vi "SEK2020v1VI5SeguirTubulacao.vi"(8 "Parâmetros":T1={"Azul Max EV3 Cor"=17, "Azul Min EV3 Cor"=0, "Verde Max EV3 Cor"=6, "Verde Min EV3 Cor"=0, "Vermelho Max Ev3 Cor"=0, "Vermelho Min EV3 Cor"=0, "Chão EV3 Cor"=0.0, "Branco Max EV3 Cor"=0.0, "Branco Min EV3 Cor"=0.0, "Preto Max EV3 Cor"=0.0, "Preto Min EV3 Cor"=0.0, "Distância Tubulação"=0.0, "Distância Frontal"=0.0, "Amarelo Max EV3 Cor"=0.0, "Amarelo Min EV3 Cor"=0.0, "Distância Lateral"=0.0, "90°"=0.0, "180°"=0.0, "Seguidor de Linha"=0.0}, 10 "NXT/EV3":T2) -> (1 "Boolean":bool, 2 "d-e":i32, 3 "NXT/EV3 2":T2)   [LabVIEW 2016]
uses:
  <vilib>/NXT/Subs/LVHSConnector.ctl
  <vilib>/NXT/LegoClasses/BrickReference/BrickReference.lvclass
  <vilib>/NXT/Block Support/NXT_OutputPort.ctl
  <vilib>/NXT/Block Support/NXT_InputPort.ctl
  <vilib>/NXT/Dual Mode Library/Sensors/EV3_Ultrasonic_CM.vi
  <vilib>/NXT/Dual Mode Library/Sensors/Touch_Pressed.vi
  <vilib>/NXT/NXTIO Xnodes/NXTIONodeSubVIs/NXTMoveMotors.vi
  <vilib>/NXT/NXTIO Xnodes/NXTIONodeSubVIs/NXTStopMotors.vi
  <vilib>/NXT/Dual Mode Library/Sensors/EV3_Color_Reflect.vi
  <vilib>/NXT/NXTIO Xnodes/AddressXNode/NXTIOAddress.xnode
  <vilib>/NXT/NXTIO Xnodes/NXTIOXNode/NXTIO.xnode
panel:
  # "Sensor EV3 Cor"
  # "Sensor Ultrassônico"
  # "Sensor Giroscópio"
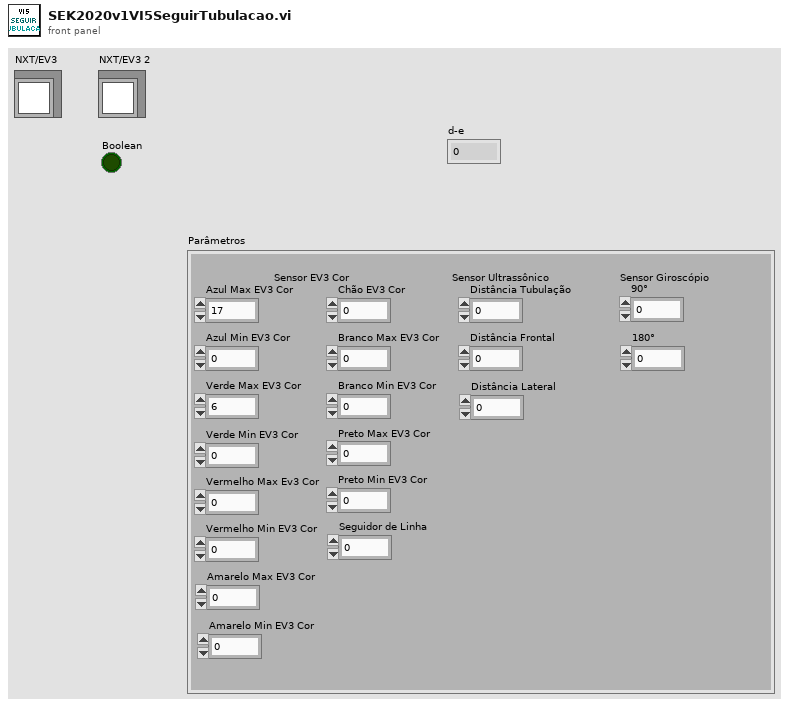
[diagram p1: front panel]
types:
  T1 = cluster{"Azul Max EV3 Cor":i32, "Azul Min EV3 Cor":i32, "Verde Max EV3 Cor":i32, "Verde Min EV3 Cor":i32, "Vermelho Max Ev3 Cor":i32, "Vermelho Min EV3 Cor":i32, "Chão EV3 Cor":sgl, "Branco Max EV3 Cor":sgl, "Branco Min EV3 Cor":sgl, "Preto Max EV3 Cor":sgl, "Preto Min EV3 Cor":sgl, "Distância Tubulação":sgl, "Distância Frontal":sgl, "Amarelo Max EV3 Cor":dbl, "Amarelo Min EV3 Cor":dbl, "Distância Lateral":sgl, "90°":sgl, "180°":sgl, "Seguidor de Linha":dbl}
  T2 = typedef "LVHSConnector.ctl" = refnum<class "BrickReference.lvclass">
  T3 = typedef "NXT_OutputPort.ctl" = u8
  T4 = typedef "NXT_InputPort.ctl" = u32
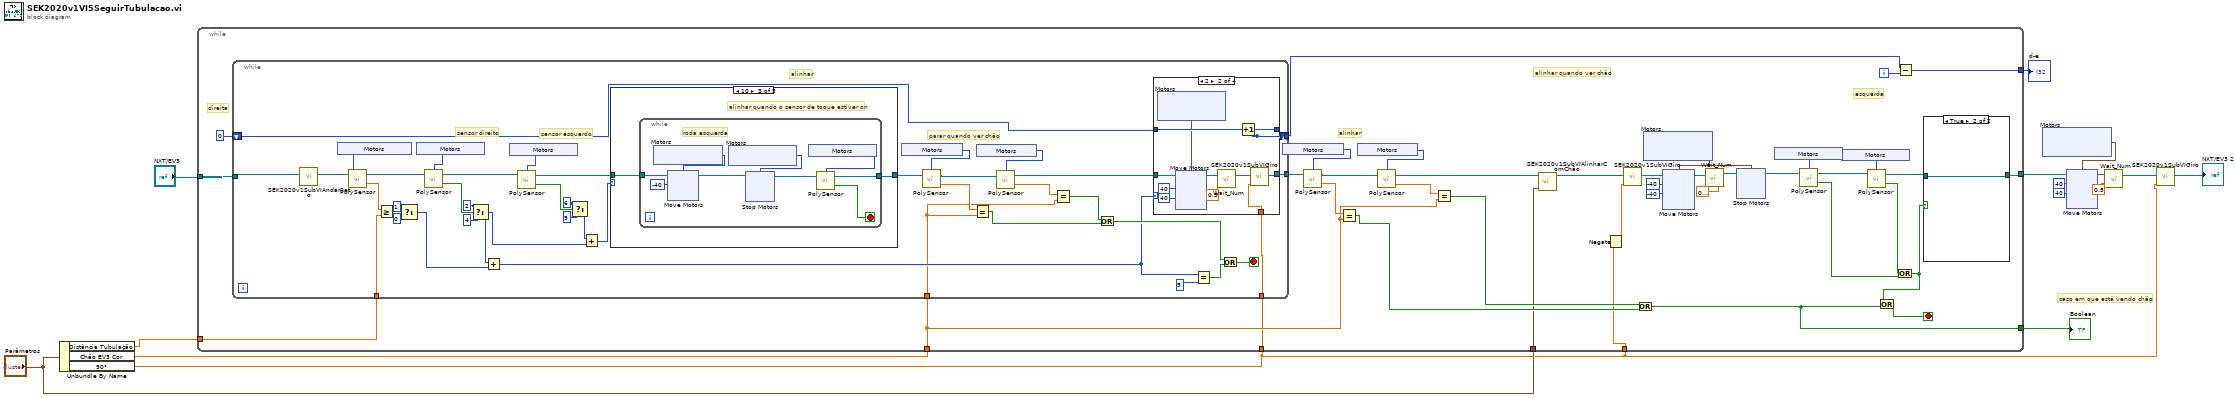
[diagram p0: block diagram]
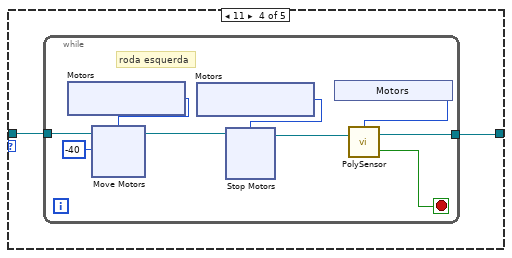
[diagram p4: hidden frame]
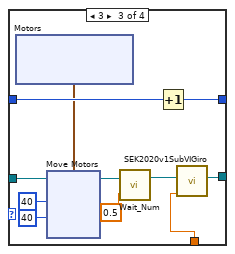
[diagram p7: hidden frame]
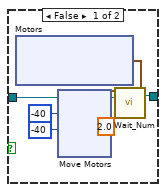
[diagram p9: hidden frame]
diagram:
  # "caso em que está vendo chão"
  n1 = Unbundle By Name("Parâmetros") -> ("Distância Tubulação"=w2:sgl, "Chão EV3 Cor"=w15:sgl, "90°"=w1:sgl)
  n2 = while {
    tunnel: "NXT/EV3" -> [w54]
    tunnel: [w33] -> w6
    tunnel: w15 -> [w39]
    tunnel: [w27] -> w13
    tunnel: [w35] -> w4
    tunnel: "Parâmetros" -> [w20]
    tunnel: w1 -> [w19]
    tunnel: w2 -> [w18]
    tunnel: w1 -> [w17]
    i -> [w37]
    stop <- w25 stop-if-true
    # "alinhar quando ver chão"
    # "esquerda"
    # "direita"
    # "alinhar"
    n3 = while {
      tunnel: w54 -> [w62]
      tunnel: [w83] -> w40
      tunnel: w39 -> [w59]
      tunnel: [w64] -> _
      shift-right: [w64] -> w36
      shift-left: 0 -> [w65]
      tunnel: w19 -> [w56]
      tunnel: w18 -> [w55]
      stop <- w66 stop-if-true
      # "parar quando ver chão"
      # "alinhar"
      # "sensor esquerdo"
      # "sensor direito"
      n4 = call "SEK2020v1SubVIAndarReto.vi"("NXT/EV3"=w62) -> ("NXT/EV3 2"=w96:T2)  [unwired: 9 in]
      n5 = xnode "Motors"() -> ("Sensor"=w95:T4)
      n6 = call-poly <vilib>:"PolySensor.vi"("NXT/EV3"=w96, "Port (Port 1)"=w95) -> ("Centimeters"=w92:sgl, "NXT/EV3"=w94:T2)  [unwired: 1 in]
      n7 = Greater Or Equal?(x=w92, y=w55) -> (x >= y?=w91:bool)
      n8 = Select(t=1, s=w91, f=0) -> (s? t:f=w85:i32)
      n9 = xnode "Motors"() -> ("Sensor"=w93:T4)
      n10 = call-poly <vilib>:"PolySensor.vi"("NXT/EV3"=w94, "Port (Port 1)"=w93) -> ("Yes / No"=w88:bool, "NXT/EV3"=w81:T2)  [unwired: 1 in]
      n11 = Select(t=2, s=w88, f=4) -> (s? t:f=w76:i32)
      n12 = Add(x=w76, y=w85) -> (x+y=w63:i32)
      n13 = xnode "Motors"() -> ("Sensor"=w82:T4)
      n14 = call-poly <vilib>:"PolySensor.vi"("NXT/EV3"=w81, "Port (Port 1)"=w82) -> ("Yes / No"=w78:bool, "NXT/EV3"=w77:T2)  [unwired: 1 in]
      n15 = Select(t=6, s=w78, f=9) -> (s? t:f=w75:i32)
      n16 = Add(x=w75, y=w76) -> (x+y=w74:i32)
      n17 = case shown="10" w74 {
        tunnel: w77 -> [w99 w100 w102 w128 w153]
        tunnel: [w99 w100 w101 w127 w153] -> w73
        frame 0, Default {
        }
        frame 8 {
        }
        frame 10 {
          # "alinhar quando o sensor de toque estiver on"
          n18 = while {
            tunnel: [w109] -> w101
            tunnel: w102 -> [w103]
            stop <- w108 stop-if-true
            # "roda esquerda"
            n19 = xnode "Motors"() -> ("Motor"=w111:T3)
            n20 = xnode "Move Motors"("Power/Speed 1"=i8 -40, "Motors"=w111, "NXT/EV3"=w103) -> ("NXT/EV3"=w106:T2)
            n21 = xnode "Motors"() -> ("Motor"=w104:T3)
            n22 = xnode "Stop Motors"("Motors"=w104, "NXT/EV3"=w106) -> ("NXT/EV3"=w105:T2)
            n23 = xnode "Motors"() -> ("Sensor"=w110:T4)
            n24 = call-poly <vilib>:"PolySensor.vi"("NXT/EV3"=w105, "Port (Port 1)"=w110) -> ("Yes / No"=w108:bool, "NXT/EV3"=w109:T2)  [unwired: 1 in]
          }
        }
        frame 11 {
          n25 = while {
            tunnel: w128 -> [w136]
            tunnel: [w134] -> w127
            stop <- w133 stop-if-true
            # "roda esquerda"
            n26 = xnode "Motors"() -> ("Motor"=w137:T3)
            n27 = xnode "Move Motors"("Power/Speed 1"=i8 -40, "Motors"=w137, "NXT/EV3"=w136) -> ("NXT/EV3"=w131:T2)
            n28 = xnode "Motors"() -> ("Motor"=w129:T3)
            n29 = xnode "Stop Motors"("Motors"=w129, "NXT/EV3"=w131) -> ("NXT/EV3"=w130:T2)
            n30 = xnode "Motors"() -> ("Sensor"=w135:T4)
            n31 = call-poly <vilib>:"PolySensor.vi"("NXT/EV3"=w130, "Port (Port 1)"=w135) -> ("Yes / No"=w133:bool, "NXT/EV3"=w134:T2)  [unwired: 1 in]
          }
        }
        frame 13 {
        }
      }
      n32 = xnode "Motors"() -> ("Sensor"=w72:T4)
      n33 = call-poly <vilib>:"PolySensor.vi"("NXT/EV3"=w73, "Port (Port 1)"=w72) -> ("Scaled Value"=w60:sgl, "NXT/EV3"=w70:T2)  [unwired: 1 in]
      n34 = Equal?(x=w60, y=w59) -> (x = y?=w57:bool)
      n35 = xnode "Motors"() -> ("Sensor"=w71:T4)
      n36 = call-poly <vilib>:"PolySensor.vi"("NXT/EV3"=w70, "Port (Port 1)"=w71) -> ("Scaled Value"=w69:sgl, "NXT/EV3"=w61:T2)  [unwired: 1 in]
      n37 = Equal?(x=w69, y=w59) -> (x = y?=w58:bool)
      n38 = Or(x=w58, y=w57) -> (x .or. y?=w67:bool)
      n39 = case shown="2" w63 {
        tunnel: [w158 w160 w180 w200] -> w83
        tunnel: w61 -> [w158 w161 w181 w200]
        tunnel: [w157 w169 w189 w199] -> w64
        tunnel: w65 -> [w157 w168 w188 w199]
        tunnel: w56 -> [_ w159 w179 _]
        frame 0, Default {
        }
        frame 2 {
          n40 = xnode "Motors"() -> ("Motor"=w164:cluster{"Port":T3, "Port":T3})
          n41 = xnode "Move Motors"("Power/Speed 2"=i8 40, "Power/Speed 1"=i8 40, "Motors"=w164, "NXT/EV3"=w161) -> ("NXT/EV3"=w165:T2)
          n42 = call <vilib>:"Wait_Num.vi"("Time (1 sec)"=sgl 0.5, "NXT/EV3"=w165) -> ("NXT/EV3"=w162:T2)  [unwired: 2 in]
          n43 = Increment(x=w168) -> (x+1=w169:i32)
          n44 = call "SEK2020v1SubVIGiro.vi"("ANGULO"=w159, "NXT/EV3"=w162) -> ("NXT/EV3 2"=w160:T2)  [unwired: 7 in]
        }
        frame 3 {
          n45 = xnode "Motors"() -> ("Motor"=w184:cluster{"Port":T3, "Port":T3})
          n46 = xnode "Move Motors"("Power/Speed 2"=i8 40, "Power/Speed 1"=i8 40, "Motors"=w184, "NXT/EV3"=w181) -> ("NXT/EV3"=w185:T2)
          n47 = call <vilib>:"Wait_Num.vi"("Time (1 sec)"=sgl 0.5, "NXT/EV3"=w185) -> ("NXT/EV3"=w182:T2)  [unwired: 2 in]
          n48 = Increment(x=w188) -> (x+1=w189:i32)
          n49 = call "SEK2020v1SubVIGiro.vi"("ANGULO"=w179, "NXT/EV3"=w182) -> ("NXT/EV3 2"=w180:T2)  [unwired: 7 in]
        }
        frame 4, 5 {
        }
      }
      n50 = Equal?(x=w63, y=5) -> (x = y?=w68:bool)
      n51 = Or(x=w67, y=w68) -> (x .or. y?=w66:bool)
    }
    n52 = xnode "Motors"() -> ("Sensor"=w45:T4)
    n53 = call-poly <vilib>:"PolySensor.vi"("NXT/EV3"=w40, "Port (Port 1)"=w45) -> ("Scaled Value"=w42:sgl, "NXT/EV3"=w43:T2)  [unwired: 1 in]
    n54 = Equal?(x=w42, y=w39) -> (x = y?=w24:bool)
    n55 = xnode "Motors"() -> ("Sensor"=w44:T4)
    n56 = call-poly <vilib>:"PolySensor.vi"("NXT/EV3"=w43, "Port (Port 1)"=w44) -> ("Scaled Value"=w41:sgl, "NXT/EV3"=w22:T2)  [unwired: 1 in]
    n57 = Equal?(x=w41, y=w39) -> (x = y?=w23:bool)
    n58 = call "SEK2020v1SubVIAlinharComChão.vi"("Parâmetros"=w20, "NXT/EV3"=w22) -> ("NXT/EV3 2"=w21:T2)  [unwired: 9 in]
    n59 = Negate(x=w17) -> (-x=w16:sgl)
    n60 = call "SEK2020v1SubVIGiro.vi"("ANGULO"=w16, "NXT/EV3"=w21) -> ("NXT/EV3 2"=w52:T2)  [unwired: 7 in]
    n61 = Or(x=w23, y=w24) -> (x .or. y?=w27:bool)
    n62 = xnode "Motors"() -> ("Motor"=w30:cluster{"Port":T3, "Port":T3})
    n63 = xnode "Move Motors"("Power/Speed 2"=i8 -40, "Power/Speed 1"=i8 -40, "Motors"=w30, "NXT/EV3"=w52) -> ("NXT/EV3"=w32:T2)
    n64 = call <vilib>:"Wait_Num.vi"("Time (1 sec)"=sgl 0.7, "NXT/EV3"=w32) -> ("NXT/EV3"=w31:T2)  [unwired: 2 in]
    n65 = xnode "Stop Motors"("Motors"=w30, "NXT/EV3"=w31) -> ("NXT/EV3"=w28:T2)
    n66 = xnode "Motors"() -> ("Sensor"=w53:T4)
    n67 = call-poly <vilib>:"PolySensor.vi"("NXT/EV3"=w28, "Port (Port 1)"=w53) -> ("Yes / No"=w47:bool, "NXT/EV3"=w48:T2)  [unwired: 1 in]
    n68 = xnode "Motors"() -> ("Sensor"=w49:T4)
    n69 = call-poly <vilib>:"PolySensor.vi"("NXT/EV3"=w48, "Port (Port 1)"=w49) -> ("Yes / No"=w46:bool, "NXT/EV3"=w34:T2)  [unwired: 1 in]
    n70 = Or(x=w46, y=w47) -> (x .or. y?=w26:bool)
    n71 = Or(x=w26, y=w27) -> (x .or. y?=w25:bool)
    n72 = Subtract(x=w36, y=w37) -> (x-y=w35:i32)
    n73 = case shown="True" w26 {
      tunnel: [w208 w224] -> w33
      tunnel: w34 -> [w209 w224]
      frame False {
        n74 = xnode "Motors"() -> ("Motor"=w211:cluster{"Port":T3, "Port":T3})
        n75 = xnode "Move Motors"("Power/Speed 2"=i8 -40, "Power/Speed 1"=i8 -40, "Motors"=w211, "NXT/EV3"=w209) -> ("NXT/EV3"=w212:T2)
        n76 = call <vilib>:"Wait_Num.vi"("Time (1 sec)"=sgl 2.0, "NXT/EV3"=w212) -> ("NXT/EV3"=w208:T2)  [unwired: 2 in]
      }
      frame True {
      }
    }
  }
  "Boolean" <- w13
  "d-e" <- w4
  n77 = xnode "Motors"() -> ("Motor"=w8:cluster{"Port":T3, "Port":T3})
  n78 = xnode "Move Motors"("Power/Speed 2"=i8 40, "Power/Speed 1"=i8 40, "Motors"=w8, "NXT/EV3"=w6) -> ("NXT/EV3"=w10:T2)
  n79 = call <vilib>:"Wait_Num.vi"("Time (1 sec)"=sgl 0.5, "NXT/EV3"=w10) -> ("NXT/EV3"=w9:T2)  [unwired: 2 in]
  n80 = call "SEK2020v1SubVIGiro.vi"("ANGULO"=w1, "NXT/EV3"=w9) -> ("NXT/EV3 2"=→"NXT/EV3 2":T2)  [unwired: 7 in]
